vi "sv_Compute Energy and Level of Tones.vi"(11 "reference tones":T1(array[cluster]) {"phase (deg)" format="%0.3p"; "amplitude [EU pk]" format="%0.3p"; "frequency [Hz]" format="%0.3p"}) -> (2 "level [EU rms]":dbl format="%_6g", 3 "energy level [EU^2 rms]":dbl format="%_6g")   [LabVIEW 2017]
panel:
  # "amplitude [EU pk]"
  # "frequency [Hz]"
  # "amplitude [EU pk]"
  # "phase [deg]"
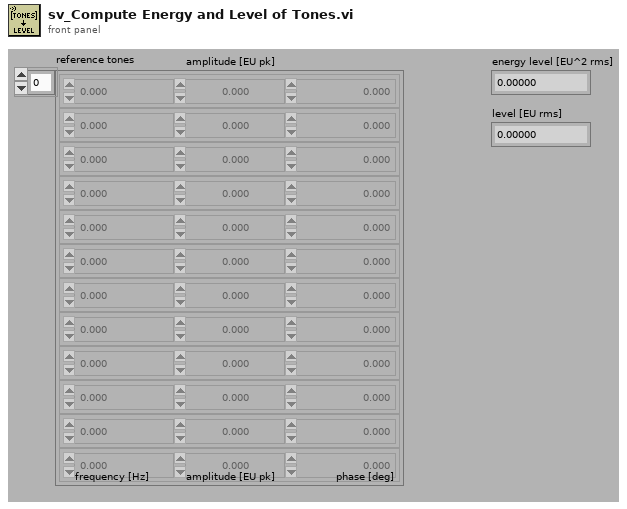
[diagram p1: front panel]
types:
  T1 = cluster{"frequency [Hz]":dbl, "amplitude [EU pk]":dbl, "phase (deg)":dbl}[]
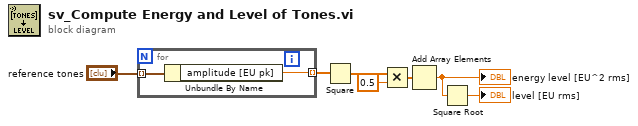
[diagram p0: block diagram]
diagram:
  n1 = for {
    tunnel: "reference tones" -> [w9] mode=indexing
    tunnel: [w8] -> w6 mode=indexing
    n2 = Unbundle By Name(w9) -> ("amplitude [EU pk]"=w8:dbl)
  }
  n3 = Square(x=w6) -> (x^2=w5:dbl[])
  n4 = Multiply(x=w5, y=0.5) -> (x*y=w3:dbl[])
  n5 = Add Array Elements(numeric array=w3) -> (sum=w1:dbl)
  "energy level [EU^2 rms]" <- w1
  n6 = Square Root(x=w1) -> (sqrt(x)=→"level [EU rms]":dbl)
